vi "Create Message VI (from Accessor).vi"(8 "error in (no error)":errorcluster, 9 "accessor type":T1="Get", 10 "rpc message name":string, 11 "rpc messages folder in":refnum<vi>) -> (0 "error out":errorcluster, 1 "created?":bool, 2 "accessor vi":refnum<vi>, 3 "rpc messages folder out":refnum<vi>)   [LabVIEW 2019, in "gRPC Template Creation Utility.lvlib"]
uses:
  gRPC Template Creation Utility.lvlib
  TypeDefs/Method Accessor Type.ctl
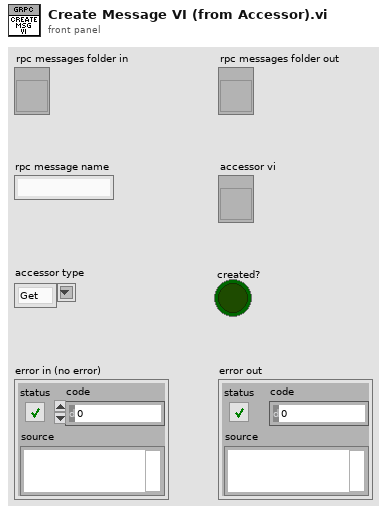
[diagram p1: front panel]
types:
  T1 = typedef "gRPC Template Creation Utility.lvlib/Method Accessor Type.ctl" = string
  T2 = enum32{"invalid VI type", "Standard VI", "Control VI", "Global VI", "Polymorphic VI", "Configuration VI", "SubSystem", "Facade VI", "Method VI"}
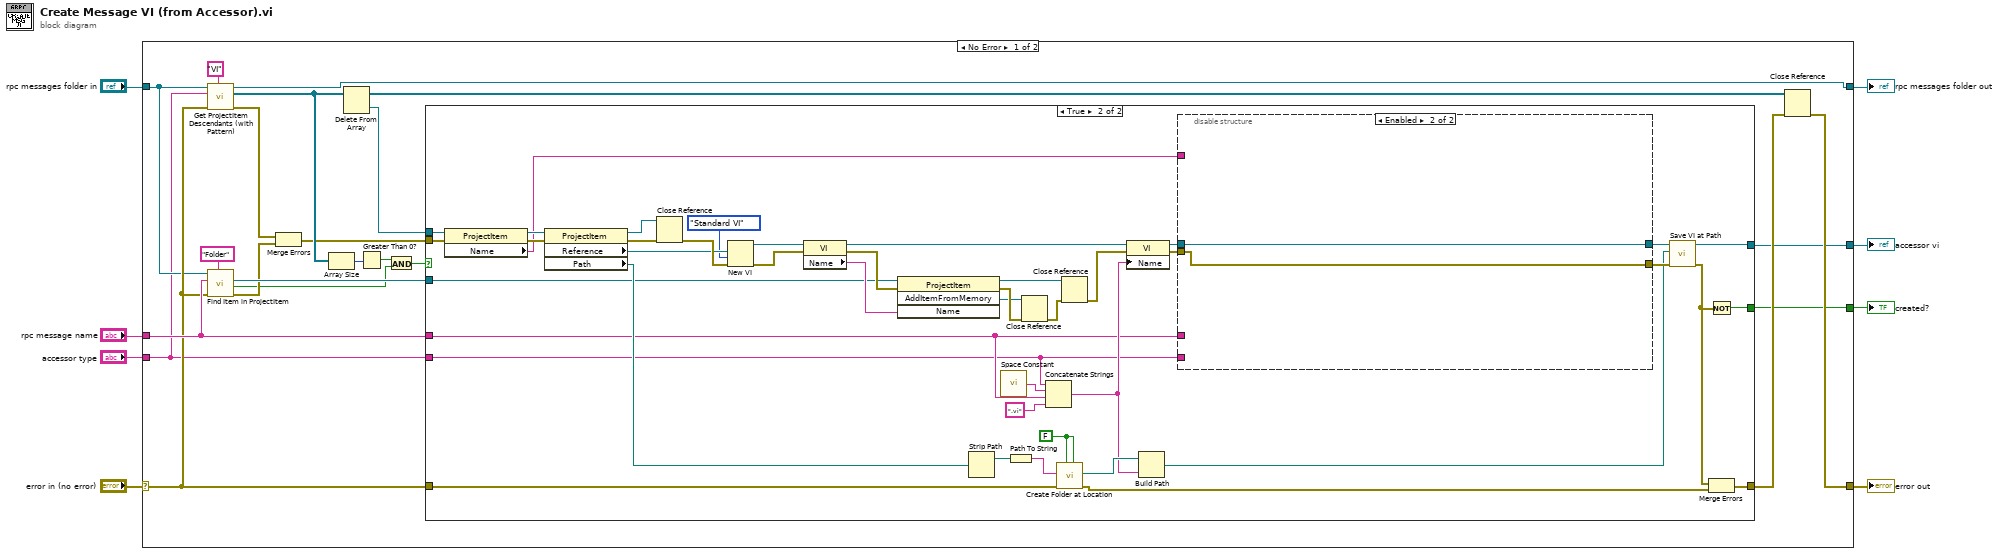
[diagram p0: block diagram]
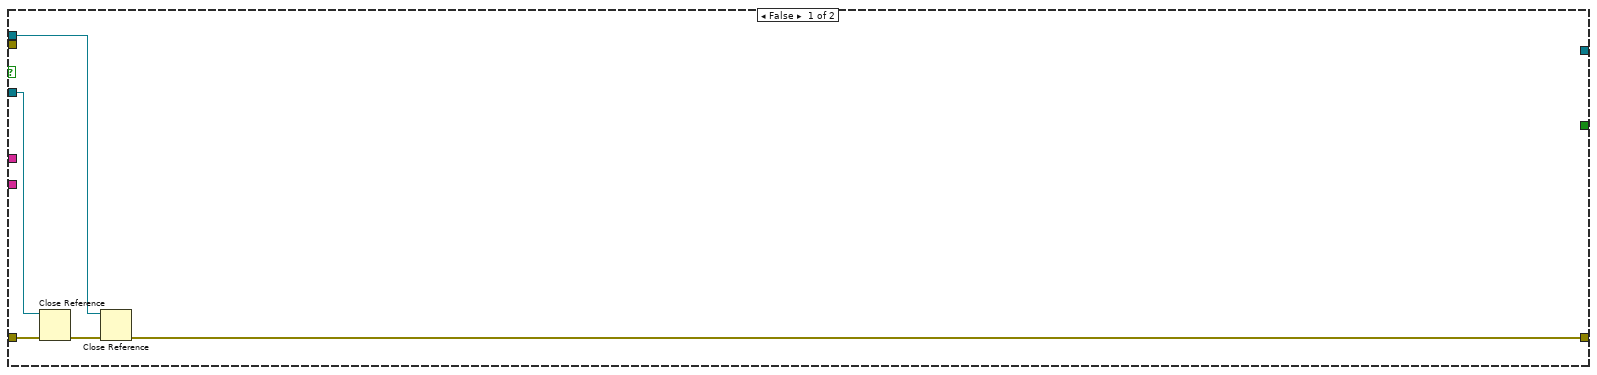
[diagram p2: hidden frame]
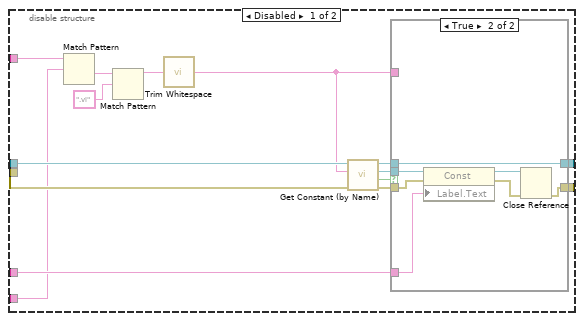
[diagram p3: hidden frame]
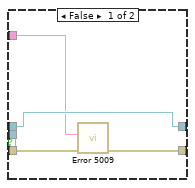
[diagram p4: hidden frame]
diagram:
  n1 = case shown="No Error" "error in (no error)" {
    selector: "error in (no error)" -> [w16 w107]
    tunnel: "rpc message name" -> [w26 _]
    tunnel: "rpc messages folder in" -> [w10 w106]
    tunnel: [w14 w107] -> w5
    tunnel: [w13 w106] -> w4
    tunnel: [w12 _] -> w3
    tunnel: [w11 _] -> w2
    tunnel: "accessor type" -> [w9 _]
    frame No Error {
      n2 = call "Get ProjectItem Descendants (with Pattern).vi"("Type"="VI", "error in (no error)"=w16, "Pattern"=w9, "ProjectItem in"=w10) -> ("error out"=w20:errorcluster, "ProjectItem descendents"=w25:refnum<vi>[], "ProjectItem out"=w13:refnum<vi>)  [unwired: 5 in]
      n3 = call "Find Item in ProjectItem.vi"("Item Type"="Folder", "error in (no error)"=w16, "Name"=w26, "ProjectItem in"=w10) -> ("error out"=w19:errorcluster, "Found ?"=w18:bool, "Item Refnum out"=w23:refnum<vi>)  [unwired: 4 in, 1 out]
      n4 = Merge Errors(w20, w19) -> (w17:errorcluster)
      n5 = Array Size(array=w25) -> (size(s)=w24:i32)
      n6 = Delete From Array(array=w25) -> (deleted portion=w28:refnum<vi>, array with subset deleted=w30:refnum<vi>[])  [unwired: 2 in]
      n7 = Greater Than 0?(x=w24) -> (x > 0?=w22:bool)
      n8 = And(x=w22, y=w18) -> (x .and. y?=w21:bool)
      n9 = case shown="True" w21 {
        tunnel: w26 -> [_ w37]
        tunnel: [w31 w74] -> w15
        tunnel: [_ w43] -> w11
        tunnel: w28 -> [w35 w50]
        tunnel: [_ w59] -> w12
        tunnel: w23 -> [w34 w55]
        tunnel: w16 -> [w33 w54]
        tunnel: w17 -> [_ w49]
        tunnel: w9 -> [_ w36]
        frame False {
          n10 = Close Reference(reference=w34, error in (no error)=w33) -> (error out=w32:errorcluster)
          n11 = Close Reference(reference=w35, error in (no error)=w32) -> (error out=w31:errorcluster)
        }
        frame True {
          w72 = FALSE ("Use Relative (F)")
          n12 = property class="ProjectItem"(reference=w50, error in=w49) -> (reference out=w48:refnum<vi>, error out=w47:errorcluster, "Name"=w38:string)
          n13 = property class="ProjectItem"(reference=w48, error in=w47) -> (reference out=w77:refnum<vi>, error out=w75:errorcluster, "Reference"=w65:refnum<vi>, "Path"=w68:path)
          n14 = Close Reference(reference=w77, error in (no error)=w75) -> (error out=w76:errorcluster)
          n15 = New VI(8:w76, 9:T2."Standard VI" ("vi type (standard vi)"), 10:w65) -> (0:w64:errorcluster, 3:w62:refnum<vi>)  [unwired: 1 in, 3 out]
          n16 = property class="VI"(reference=w62, error in=w64) -> (reference out=w69:refnum<vi>, error out=w70:errorcluster, "Name"=w66:string)
          n17 = invoke class="ProjectItem" method="AddItemFromMemory"(reference=w55, error in=w70, "Name"=w66) -> (reference out=w61:refnum<vi>, error out=w53:errorcluster, "AddItemFromMemory"=w52:refnum<vi>)  [unwired: 1 in, 1 out]
          n18 = Strip Path(path=w68) -> (stripped path=w39:path)  [unwired: 1 out]
          n19 = call <vilib>:"Space Constant.vi"() -> ("String"=w58:string)
          n20 = Path To String(path=w39) -> (string=w67:string)
          n21 = Close Reference(reference=w52, error in (no error)=w53) -> (error out=w51:errorcluster)
          n22 = Concatenate Strings(w36, w58, w37, ".vi" ("string")) -> (w56:string)
          n23 = call "Create Folder at Location.vi"("Override existing (F)"=w72, "Use Relative (F)"=w72, "Error In"=w54, "Path"=w67) -> ("Error Out"=w73:errorcluster, "Full path out"=w71:path)  [unwired: 5 in, 1 out]
          n24 = Close Reference(reference=w61, error in (no error)=w51) -> (error out=w60:errorcluster)
          n25 = property class="VI"(reference=w69, error in=w60, "Name"=w56) -> (reference out=w46:refnum<vi>, error out=w45:errorcluster)
          n26 = Build Path(base path=w71, name or relative path=w56) -> (appended path=w42:path)
          n27 = disable-structure shown="Enabled" {
            disable-tunnel: w46 -> [w91 w105]
            disable-tunnel: w45 -> [w90 w104]
            disable-tunnel: w37 -> [w89 _]
            disable-tunnel: [w87 w104] -> w44
            disable-tunnel: [w84 w105] -> w40
            disable-tunnel: w38 -> [w80 _]
            disable-tunnel: w36 -> [w78 _]
            frame Disabled {
              n28 = Match Pattern(string=w80, regular expression=w78) -> (after substring=w82:string)  [unwired: 1 in, 3 out]
              n29 = Match Pattern(string=w82, regular expression=".vi") -> (before substring=w83:string)  [unwired: 1 in, 3 out]
              n30 = call <vilib>:"Trim Whitespace.vi"("string"=w83) -> ("trimmed string"=w79:string)  [unwired: 1 in]
              n31 = call "Get Constant (by Name).vi"("error in (no error)"=w90, "Constant Label"=w79, "Owner VI in"=w91) -> ("error out"=w88:errorcluster, "Found ?"=w86:bool, "Const ref out"=w92:refnum<vi>, "Owner VI out"=w85:refnum<vi>)  [unwired: 5 in]
              n32 = case shown="True" w86 {
                tunnel: w92 -> [_ w103]
                tunnel: w89 -> [_ w102]
                tunnel: w88 -> [w95 w101]
                tunnel: [w94 w98] -> w87
                tunnel: w85 -> [w96 w97]
                tunnel: [w96 w97] -> w84
                tunnel: w79 -> [w93 _]
                frame False {
                  n33 = call "Error 5009.vi"("error in (no error)"=w95, "Cluster Definition Constant"=w93) -> ("error out"=w94:errorcluster)  [unwired: 9 in]
                }
                frame True {
                  n34 = property class="Const"(reference=w103, error in=w101, "Label.Text"=w102) -> (reference out=w100:refnum<vi>, error out=w99:errorcluster)
                  n35 = Close Reference(reference=w100, error in (no error)=w99) -> (error out=w98:errorcluster)
                }
              }
            }
            frame Enabled {
            }
          }
          n36 = call "Save VI at Path.vi"("error in (no error)"=w44, "Path"=w42, "VI in"=w40) -> ("error out"=w41:errorcluster, "VI out"=w43:refnum<vi>)  [unwired: 6 in, 1 out]
          n37 = Not(x=w41) -> (.not. x?=w59:bool)
          n38 = Merge Errors(w41, w73) -> (w74:errorcluster)
        }
      }
      n39 = Close Reference(reference=w30, error in (no error)=w15) -> (error out=w14:errorcluster)
    }
    frame Error {
    }
  }
  "error out" <- w5
  "rpc messages folder out" <- w4
  "created?" <- w3
  "accessor vi" <- w2
